vi "Line Configuration Dialog.vi"(8 "error in":errorcluster, 9 "engine configuration in":refnum<class "engine configuration.lvclass">, 10 "tag bus configurable plugin module configuration":refnum<class "Scan Engine configuration.lvclass">, 11 "Line":T4) -> (0 "error out":errorcluster, 1 "success":bool, 2 "changed":bool, 3 "Mappings out":T3)   [LabVIEW 2015, in "Scan Engine editor node.lvclass"]
uses:
  <vilib>/NI/DCAF/Modules/scan engine/editor node/Scan Engine editor node.lvclass
  <vilib>/NI/DCAF/Modules/scan engine/configuration/Scan Engine configuration.lvclass
  <vilib>/NI/Tag Bus/tag/tag descriptor.lvclass
  <vilib>/NI/Module Execution Interface/Engine Configuration/engine configuration.lvclass
  <vilib>/NI/Tag Bus Module Framework/channel/TBM channel.lvclass
  <vilib>/NI/DCAF/Modules/scan engine/configuration/Line.ctl
  <vilib>/NI/DCAF/Modules/scan engine/editor node/Map.ctl
  <vilib>/NI/DCAF/Modules/scan engine/editor node/Mappings.ctl
  <vilib>/NI/DCAF UI Toolkit/Controls/DCAF UI Elements.lvlib
  <vilib>/NI/DCAF/Modules/scan engine/configuration/permissions.ctl
  <vilib>/NI/DCAF/Modules/scan engine/configuration/Protocol.ctl
panel:
  in  "Variable Name":string
  in  "Protocol":T1
  out "errors":string
  in  "Access Type":T2
  in  "Tag":i32(listbox)
  in  "Data Type":i32(listbox)
  in  "hostname":string
  in  "cancel":bool
  in  "ok":bool
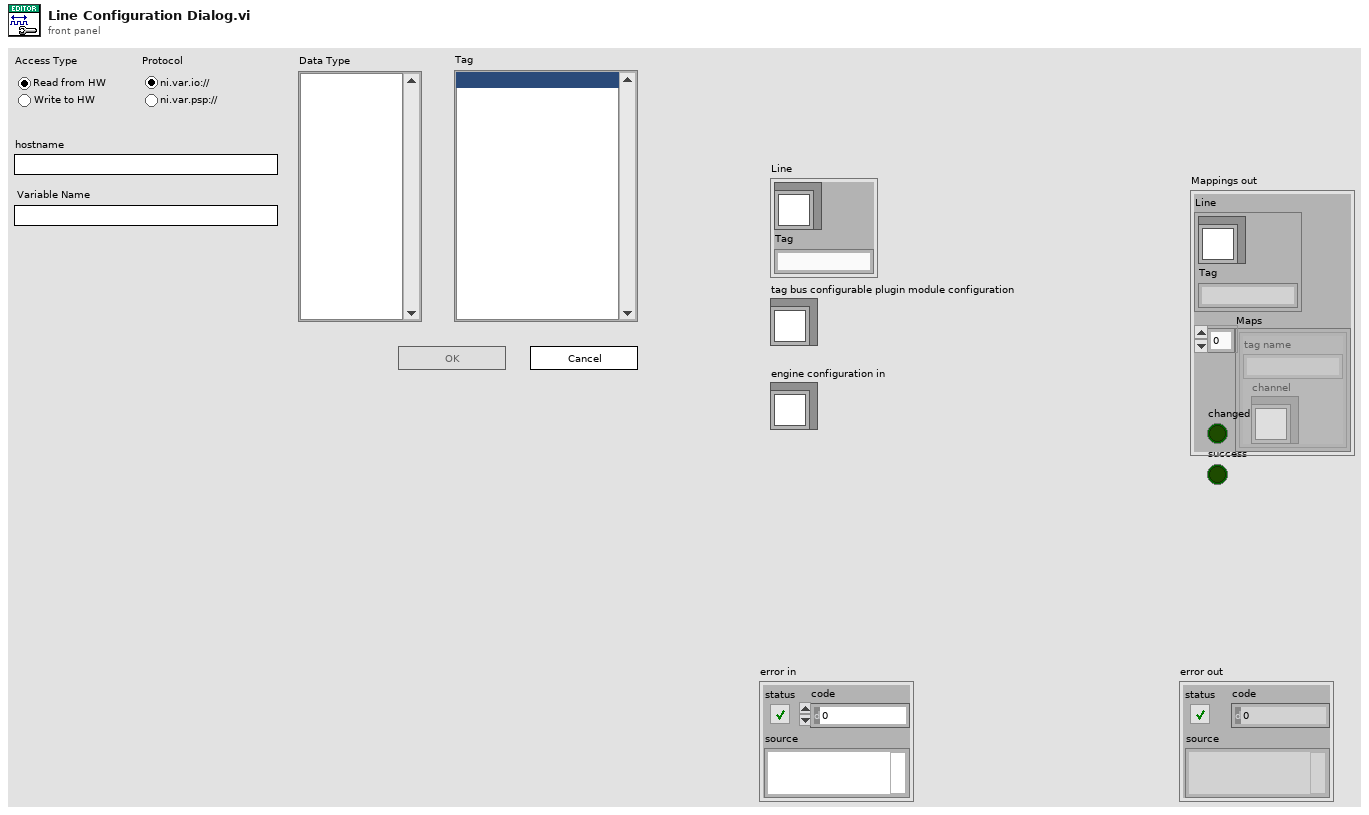
[diagram p1: front panel]
types:
  T1 = typedef "Scan Engine configuration.lvclass/Protocol.ctl" = enum32{"ni.var.io://", "ni.var.psp://"}
  T2 = typedef "Scan Engine configuration.lvclass/permissions.ctl" = enum32{"Read from HW", "Write to HW"}
  T3 = typedef "Scan Engine editor node.lvclass/Mappings.ctl" = cluster{"Line":T4, "Maps":T5[]}
  T4 = typedef "Scan Engine configuration.lvclass/Line.ctl" = cluster{"channel":refnum<class "TBM channel.lvclass">, "Tag":string}
  T5 = typedef "Scan Engine editor node.lvclass/Map.ctl" = cluster{"channel":refnum<class "TBM channel.lvclass">, "tag name":string}
  T6 = typedef "tag bus.lvlib/tag descriptor.lvclass/Data Type.ctl" = enum16{"Double", "Single", "I64", "I32", "I16", "I8", "U64", "U32", "U16", "U8", "Boolean", "String", "Array of Double", "Array of Single", "Array of I64", "Array of I32", "Array of I16", "Array of I8", "Array of U64", "Array of U32", "Array of U16", "Array of U8", "Array of Boolean", "Array of String"}
  T7 = typedef "TBM channel.lvclass/channel classification.ctl" = enum16{"input data", "output data", "processing parameter", "processing result"}
  T8 = typedef "Scan Engine editor node.lvclass/permissions.ctl" = enum32{"Read from HW", "Write to HW"}
  T9 = enum8{"Enabled", "Disabled", "Disabled and Grayed Out"}
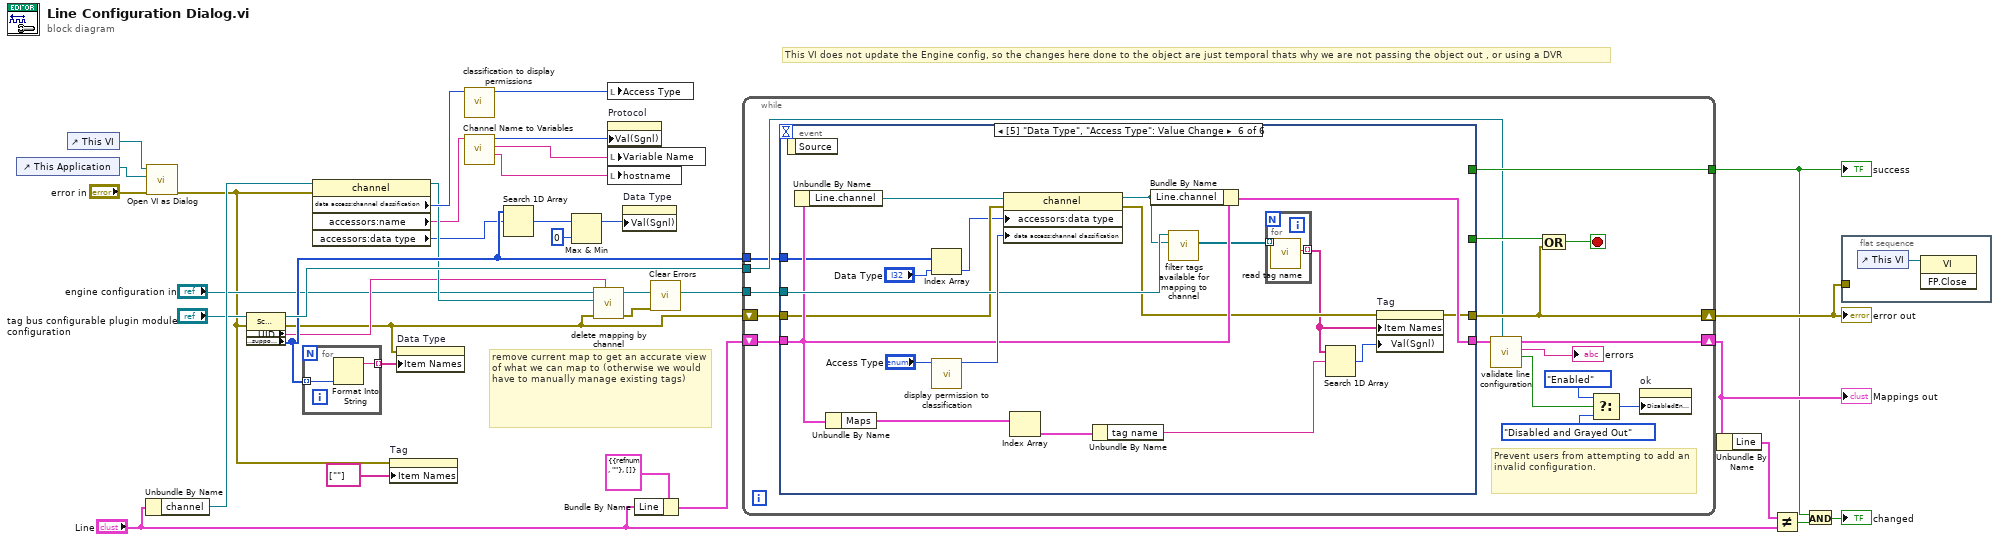
[diagram p0: block diagram]
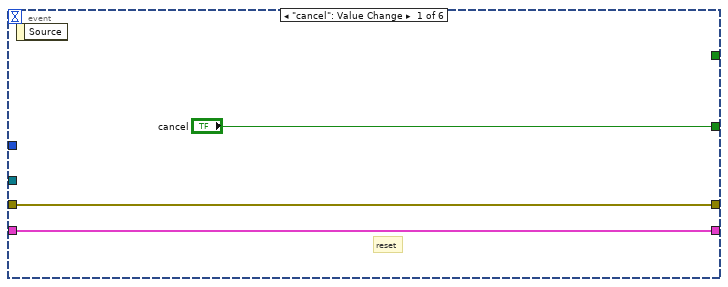
[diagram p2: hidden frame]
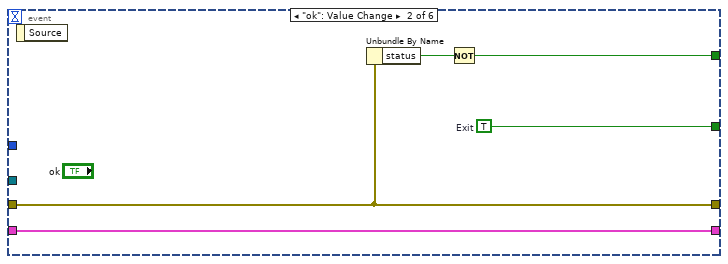
[diagram p3: hidden frame]
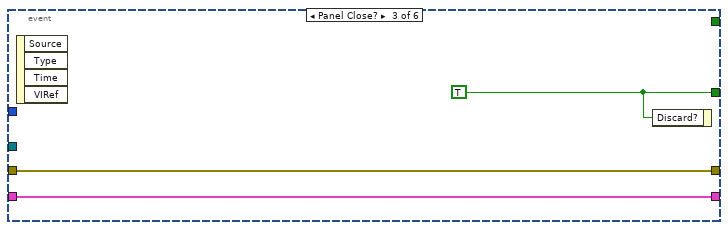
[diagram p4: hidden frame]
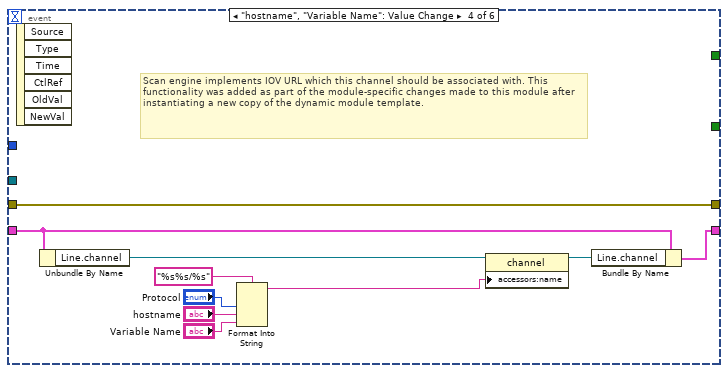
[diagram p5: hidden frame]
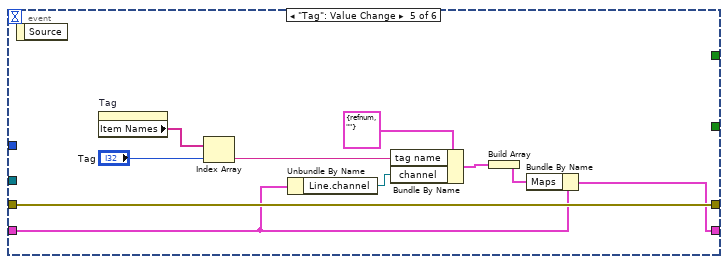
[diagram p6: hidden frame]
diagram:
  # "This VI does not update the Engine config, so the changes here done to the object are just temporal thats why we are not passing the object out , or using a DVR"
  # "remove current map to get an accurate view of what we can map to (otherwise we would have to manually manage existing tags)"
  n1 = control-ref of="This Application"() -> (w9:refnum<vi>)
  n2 = control-ref of="This VI"() -> (w10:refnum<vi>)
  n3 = Unbundle By Name("Line") -> ("channel"=w30:refnum<class "TBM channel.lvclass">)
  n4 = call <vilib>:"Open VI as Dialog.vi"("error in (no error)"="error in", "This Application"=w9, "VI in"=w10) -> ("error out"=w11:errorcluster)  [unwired: 8 in]
  n5 = property class="Scan Engine configuration"(reference="tag bus configurable plugin module configuration", error in=w11) -> (reference out=w34:refnum<class "Scan Engine configuration.lvclass">, error out=w22:errorcluster, "Properties:UID"=w28:string, "Customize:Properties:supported types"=w33:T6[])
  n6 = for {
    tunnel: w33 -> [w37] mode=indexing
    tunnel: [w36] -> w27 mode=indexing
    n7 = Format Into String(w37) -> (resulting string=w36:string)  [unwired: 3 in, 1 out]
  }
  n8 = property class="channel"(reference=w30, error in=w11) -> (reference out=w29:refnum<class "TBM channel.lvclass">, "data access:channel classification"=w31:T7, "accessors:name"=w16:string, "accessors:data type"=w25:T6)  [unwired: 1 out]
  n9 = property on="Tag" class="LstBox (strict)"(error in=w11, "Item Names"=string[] [""]) -> ()  [unwired: 1 in, 2 out]
  n10 = property on="Data Type" class="LstBox (strict)"(error in=w22, "Item Names"=w27) -> ()  [unwired: 1 in, 2 out]
  n11 = call <vilib>:"classification to display permissions.vi"("channel classification"=w31) -> ("permissions"=w5:T8)  [unwired: 10 in]
  n12 = call <vilib>:"Channel Name to Variables.vi"("Channel Name"=w16) -> ("hostname"=w15:string, "Variable Name"=w14:string, "Protocol"=w13:T1)  [unwired: 8 in]
  n13 = Search 1D Array(1D array=w33, element=w25) -> (index of element=w7:i32)  [unwired: 1 in]
  n14 = Max & Min(x=w7, y=0 ("f")) -> (max(x,y)=w6:i32)  [unwired: 1 out]
  n15 = call <vilib>:"delete mapping by channel.vi"("owner ID"=w28, "error in"=w22, "channel"=w29, "engine configuration in"="engine configuration in") -> ("error out"=w24:errorcluster, "engine configuration out"=w35:refnum<class "engine configuration.lvclass">)  [unwired: 6 in]
  n16 = local write "Access Type"(w5) -> ()
  n17 = property on="Protocol" class="RadioBtnsControl (strict)"("Val(Sgnl)"=w13) -> ()  [unwired: 2 in, 2 out]
  n18 = local write "Variable Name"(w14) -> ()
  n19 = local write "hostname"(w15) -> ()
  n20 = property on="Data Type" class="LstBox (strict)"("Val(Sgnl)"=w6) -> ()  [unwired: 2 in, 2 out]
  n21 = Bundle By Name(cluster=T3 {"Line"={"channel"=refnum, "Tag"=""}, "Maps"=[]} ("Mappings out"), "Line"="Line") -> (w19:T3)
  n22 = call <vilib>:"Clear Errors.vi"("error in (no error)"=w24) -> ()  [unwired: 5 in, 2 out]
  n23 = while {
    shift-right: [w45] -> w32
    shift-left: w22 -> [w52]
    tunnel: [w51] -> w2
    shift-right: [w46] -> w17
    shift-left: w19 -> [w48]
    tunnel: w35 -> [w53]
    tunnel: w34 -> [w40]
    tunnel: w33 -> [w39]
    stop <- w49 stop-if-true
    # "Prevent users from attempting to add an invalid configuration."
    n24 = event shown="[5] \"Data Type\", \"Access Type\": Value Change" {
      selector: _ -> [_ _ _ _ _ _]
      dyn-events: _ -> [_ _ _ _ _ _]
      timeout: _ -> [_ _ _ _ _ _]
      tunnel: w53 -> [_ _ _ _ _ w101]
      tunnel: w52 -> [w56 w59 w64 w74 w84 w95]
      tunnel: [w56 w59 w64 w74 w84 w90] -> w45
      tunnel: [_ w57 _ _ _ _] -> w51
      tunnel: ["cancel" w60 w62 _ _ _] -> w50
      tunnel: w48 -> [w54 w61 w63 w72 w78 w99]
      tunnel: [w54 w61 w63 w73 w75 w98] -> w47
      tunnel: w39 -> [_ _ _ _ _ w94]
      event "cancel": Value Change {
        # "reset"
        n25 = event-data() -> ()  [unwired: 1 in, 1 out]
      }
      event "ok": Value Change {
        w60 = TRUE  # Exit
        n26 = event-data() -> ()  [unwired: 1 in, 1 out]
        n27 = Unbundle By Name(w59) -> ("status"=w58:bool)
        n28 = Not(x=w58) -> (.not. x?=w57:bool)
      }
      event Panel Close? {
        w62 = TRUE ("cancel")
        n29 = event-data() -> ()  [unwired: 1 in, 4 out]
        n30 = event-data("Discard?"=w62) -> ()  [unwired: 1 in, 1 out]
      }
      event "hostname", "Variable Name": Value Change {
        # "Scan engine implements IOV URL which this channel should be associated with. This functionality was added as part of the module-specific changes made to this module after instantiating a new copy of the dynamic module template."
        n31 = event-data() -> ()  [unwired: 1 in, 6 out]
        n32 = Unbundle By Name(w72) -> ("Line.channel"=w71:refnum<class "TBM channel.lvclass">)
        n33 = Format Into String(format string="%s%s/%s", "Protocol", "hostname", "Variable Name") -> (resulting string=w65:string)  [unwired: 2 in, 1 out]
        n34 = property class="channel"(reference=w71, "accessors:name"=w65) -> (reference out=w70:refnum<class "TBM channel.lvclass">)  [unwired: 1 in, 1 out]
        n35 = Bundle By Name(cluster=w72, "Line.channel"=w70) -> (w73:T3)
      }
      event "Tag": Value Change {
        n36 = event-data() -> ()  [unwired: 1 in, 1 out]
        n37 = property on="Tag" class="LstBox (strict)"() -> ("Item Names"=w82:string[])  [unwired: 2 in, 2 out]
        n38 = Index Array(array=w82, index="Tag") -> (element=w81:string)
        n39 = Unbundle By Name(w78) -> ("Line.channel"=w79:refnum<class "TBM channel.lvclass">)
        n40 = Bundle By Name(cluster=T5 {"channel"=refnum, "tag name"=""} ("Map"), "tag name"=w81, "channel"=w79) -> (w77:T5)
        n41 = Build Array(w77) -> (w76:T5[])
        n42 = Bundle By Name(cluster=w78, "Maps"=w76) -> (w75:T3)
      }
      event "Data Type": Value Change {
        n43 = event-data() -> ()  [unwired: 1 in, 1 out]
        n44 = Unbundle By Name(w99) -> ("Line.channel"=w103:refnum<class "TBM channel.lvclass">)
        n45 = Unbundle By Name(w99) -> ("Maps"=w87:T5[])
        n46 = Index Array(array=w94, index="Data Type") -> (element=w92:T6)
        n47 = call <vilib>:"display permission to classification.vi"("display permissions"="Access Type") -> ("channel classification"=w102:T7)  [unwired: 10 in]
        n48 = property class="channel"(reference=w103, error in=w95, "accessors:data type"=w92, "data access:channel classification"=w102) -> (reference out=w100:refnum<class "TBM channel.lvclass">, error out=w91:errorcluster)
        n49 = Index Array(array=w87) -> (element=w86:T5)  [unwired: 1 in]
        n50 = Unbundle By Name(w86) -> ("tag name"=w85:string)
        n51 = Bundle By Name(cluster=w99, "Line.channel"=w100) -> (w98:T3)
        n52 = call-dynamic "filter tags available for mapping to channel.vi"("channel to map to"=w100, "engine configuration in"=w101) -> ("filtered tags"=w97:refnum<class "tag descriptor.lvclass">[])  [unwired: 8 in, 1 out]
        n53 = for {
          tunnel: w97 -> [w105] mode=indexing
          tunnel: [w104] -> w89 mode=indexing
          n54 = call <vilib>:"read tag name.vi"("system tag in"=w105) -> ("name"=w104:string)  [unwired: 8 in, 2 out]
        }
        n55 = Search 1D Array(1D array=w89, element=w85) -> (index of element=w88:i32)  [unwired: 1 in]
        n56 = property on="Tag" class="LstBox (strict)"(error in=w91, "Item Names"=w89, "Val(Sgnl)"=w88) -> (error out=w90:errorcluster)  [unwired: 1 in, 1 out]
      }
    }
    n57 = call <vilib>:"validate line configuration.vi"("module"=w40, "Mappings in"=w47) -> ("valid?"=w44:bool, "errors"=→"errors":string, "Mappings out"=w46:T3)  [unwired: 7 in]
    n58 = Compound Arithmetic op=OR(w50, w45) -> (w49:bool)
    n59 = Select(t=T9."Enabled" ("Disabled"), s=w44, f=T9."Disabled and Grayed Out") -> (s? t:f=w41:T9)
    n60 = property on="ok" class="Bool"("DisabledEnum"=w41) -> ()  [unwired: 2 in, 2 out]
  }
  "error out" <- w32
  "success" <- w2
  "Mappings out" <- w17
  n61 = Unbundle By Name(w17) -> ("Line"=w18:T4)
  n62 = Not Equal?(x=w18, y="Line") -> (x != y?=w3:bool)
  n63 = And(x=w2, y=w3) -> (x .and. y?=→"changed":bool)
  n64 = flat-sequence {
    tunnel: w32 -> [_]
    frame #0 {
      n65 = control-ref of="This VI"() -> (w106:refnum<vi>)
      n66 = invoke class="VI" method="FP.Close"(reference=w106) -> ()  [unwired: 2 in, 3 out]
    }
  }
